vi "macro_AngleStats_AngleResidual_CallbackHelp.vi"   [LabVIEW 2019, in "Trajectory_Library.lvlib"]
uses:
  Trajectory_Library.lvlib
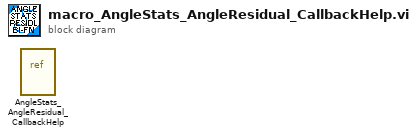
[diagram p0: block diagram]
diagram:
  n1 = vi-ref "AngleStats_AngleResidual_CallbackHelp.vi"() -> ()  [unwired: 1 out]
